vi "RT_mem_i20(SubVI).vi"(8 "Ini_val":dbl, 10 "start":bool, 11 "In":dbl format="%#_13g") -> (1 "in_vec":dbl[](array[numeric]), 3 "in_i20":dbl)   [LabVIEW 2017]
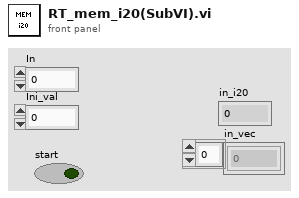
[diagram p1: front panel]
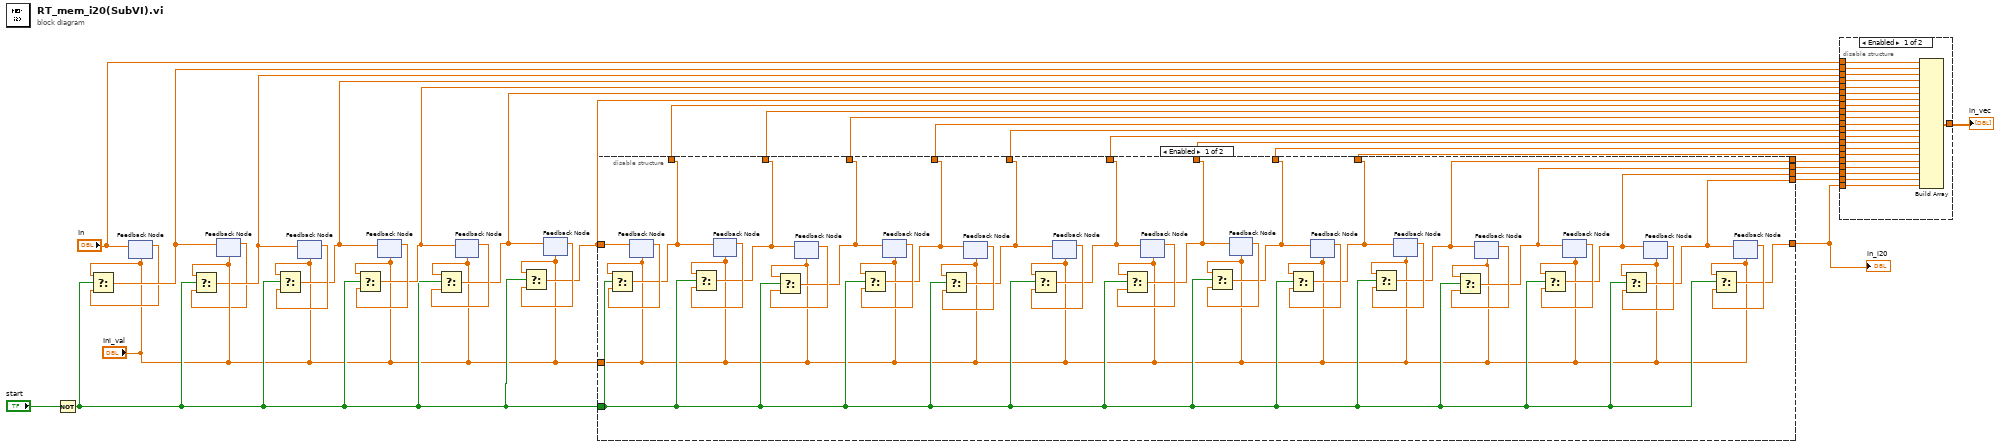
[diagram p0: block diagram]
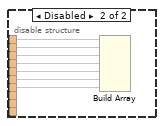
[diagram p2: hidden frame]
diagram:
  n1 = Not(x="start") -> (.not. x?=w4:bool)
  n2 = feedback #1("Ini_val") -> (w5:dbl)
  n3 = Select(t="Ini_val", s=w4, f=w5) -> (s? t:f=w6:dbl)
  n4 = feedback-in #1("In") -> ()
  n5 = feedback #2("Ini_val") -> (w1:dbl)
  n6 = Select(t="Ini_val", s=w4, f=w1) -> (s? t:f=w2:dbl)
  n7 = feedback-in #2(w6) -> ()
  n8 = feedback #3("Ini_val") -> (w28:dbl)
  n9 = Select(t="Ini_val", s=w4, f=w28) -> (s? t:f=w27:dbl)
  n10 = feedback-in #3(w2) -> ()
  n11 = feedback #4("Ini_val") -> (w29:dbl)
  n12 = Select(t="Ini_val", s=w4, f=w29) -> (s? t:f=w26:dbl)
  n13 = feedback-in #4(w27) -> ()
  n14 = feedback #5("Ini_val") -> (w30:dbl)
  n15 = Select(t="Ini_val", s=w4, f=w30) -> (s? t:f=w25:dbl)
  n16 = feedback-in #5(w26) -> ()
  n17 = feedback #6("Ini_val") -> (w31:dbl)
  n18 = Select(t="Ini_val", s=w4, f=w31) -> (s? t:f=w24:dbl)
  n19 = feedback-in #6(w25) -> ()
  n20 = disable-structure shown="Enabled" {
    disable-tunnel: w24 -> [w48 w63]
    disable-tunnel: [w47 _] -> w23
    disable-tunnel: [w46 _] -> w22
    disable-tunnel: [w45 _] -> w21
    disable-tunnel: [w44 _] -> w20
    disable-tunnel: [w43 _] -> w19
    disable-tunnel: [w42 _] -> w18
    disable-tunnel: [w41 _] -> w17
    disable-tunnel: [w40 _] -> w16
    disable-tunnel: [w39 _] -> w15
    disable-tunnel: [w38 _] -> w14
    disable-tunnel: [w37 _] -> w13
    disable-tunnel: [w36 _] -> w12
    disable-tunnel: [w35 _] -> w11
    disable-tunnel: [w34 w63] -> w10
    disable-tunnel: w4 -> [w33 _]
    disable-tunnel: "Ini_val" -> [w32 _]
    frame Enabled {
      n21 = feedback #7(w32) -> (w50:dbl)
      n22 = Select(t=w32, s=w33, f=w50) -> (s? t:f=w47:dbl)
      n23 = feedback-in #7(w48) -> ()
      n24 = feedback #8(w32) -> (w49:dbl)
      n25 = Select(t=w32, s=w33, f=w49) -> (s? t:f=w46:dbl)
      n26 = feedback-in #8(w47) -> ()
      n27 = feedback #9(w32) -> (w54:dbl)
      n28 = Select(t=w32, s=w33, f=w54) -> (s? t:f=w45:dbl)
      n29 = feedback-in #9(w46) -> ()
      n30 = feedback #10(w32) -> (w51:dbl)
      n31 = Select(t=w32, s=w33, f=w51) -> (s? t:f=w44:dbl)
      n32 = feedback-in #10(w45) -> ()
      n33 = feedback #11(w32) -> (w52:dbl)
      n34 = Select(t=w32, s=w33, f=w52) -> (s? t:f=w43:dbl)
      n35 = feedback-in #11(w44) -> ()
      n36 = feedback #12(w32) -> (w53:dbl)
      n37 = Select(t=w32, s=w33, f=w53) -> (s? t:f=w42:dbl)
      n38 = feedback-in #12(w43) -> ()
      n39 = feedback #13(w32) -> (w62:dbl)
      n40 = Select(t=w32, s=w33, f=w62) -> (s? t:f=w41:dbl)
      n41 = feedback-in #13(w42) -> ()
      n42 = feedback #14(w32) -> (w59:dbl)
      n43 = Select(t=w32, s=w33, f=w59) -> (s? t:f=w40:dbl)
      n44 = feedback-in #14(w41) -> ()
      n45 = feedback #15(w32) -> (w60:dbl)
      n46 = Select(t=w32, s=w33, f=w60) -> (s? t:f=w39:dbl)
      n47 = feedback-in #15(w40) -> ()
      n48 = feedback #16(w32) -> (w61:dbl)
      n49 = Select(t=w32, s=w33, f=w61) -> (s? t:f=w38:dbl)
      n50 = feedback-in #16(w39) -> ()
      n51 = feedback #17(w32) -> (w55:dbl)
      n52 = Select(t=w32, s=w33, f=w55) -> (s? t:f=w37:dbl)
      n53 = feedback-in #17(w38) -> ()
      n54 = feedback #18(w32) -> (w58:dbl)
      n55 = Select(t=w32, s=w33, f=w58) -> (s? t:f=w36:dbl)
      n56 = feedback-in #18(w37) -> ()
      n57 = feedback #19(w32) -> (w57:dbl)
      n58 = Select(t=w32, s=w33, f=w57) -> (s? t:f=w35:dbl)
      n59 = feedback-in #19(w36) -> ()
      n60 = feedback #20(w32) -> (w56:dbl)
      n61 = Select(t=w32, s=w33, f=w56) -> (s? t:f=w34:dbl)
      n62 = feedback-in #20(w35) -> ()
    }
    frame Disabled {
    }
  }
  "in_i20" <- w10
  n63 = disable-structure shown="Enabled" {
    disable-tunnel: w27 -> [w85 w89]
    disable-tunnel: w26 -> [w84 w88]
    disable-tunnel: w25 -> [w83 w87]
    disable-tunnel: w24 -> [w82 w86]
    disable-tunnel: w23 -> [w81 _]
    disable-tunnel: w22 -> [w80 _]
    disable-tunnel: w21 -> [w79 _]
    disable-tunnel: w20 -> [w78 _]
    disable-tunnel: w19 -> [w77 _]
    disable-tunnel: w18 -> [w76 _]
    disable-tunnel: w17 -> [w75 _]
    disable-tunnel: w16 -> [w74 _]
    disable-tunnel: w15 -> [w73 _]
    disable-tunnel: w14 -> [w72 _]
    disable-tunnel: w13 -> [w71 _]
    disable-tunnel: w12 -> [w70 _]
    disable-tunnel: w11 -> [w69 _]
    disable-tunnel: w10 -> [w68 _]
    disable-tunnel: [w67 _] -> w9
    disable-tunnel: "In" -> [w66 w92]
    disable-tunnel: w6 -> [w65 w91]
    disable-tunnel: w2 -> [w64 w90]
    frame Enabled {
      n64 = Build Array(w66, w65, w64, w85, w84, w83, w82, w81, w80, w79, w78, w77, w76, w75, w74, w73, w72, w71, w70, w69, w68) -> (w67:dbl[])
    }
    frame Disabled {
      n65 = Build Array(w92, w91, w90, w89, w88, w87, w86) -> ()  [unwired: 1 out]
    }
  }
  "in_vec" <- w9
